vi "Metro rossa data processing.vi"() -> ()   [LabVIEW 2024]
uses:
  <vilib>/Analysis/2dsp.llb/Integral Method.ctl
  <vilib>/Analysis/8numeric.llb/1D Numeric Integration.vi
  <vilib>/Utility/file.llb/Read Delimited Spreadsheet (DBL).vi
  <vilib>/express/express analysis/Spectral/Block/exnSpectralBlock spectral measurements peak poly.vi
  <vilib>/express/express analysis/Spectral/Block/exnSpectralBlock spectral measurements peak WFM.vi
  <vilib>/express/express analysis/Spectral/Block/exnSpectralBlock spectral measurements peak DDT.vi
  <vilib>/express/express analysis/Spectral/XNode/ExpressSpectralMeasurementsBlockNode.xnode
  <vilib>/Analysis/NI_AALPro.lvlib
panel:
  out "VDV integral":dbl
  out "Angle around the choosen axis":dbl[](array[numeric])
  out "Angles":waveform(dbl)(graph)
  out "Angles in frequency domain":cluster{"f0":dbl, "df":dbl, "magnitude":dbl[]}(graph)
  out "Mean angle":dbl
  out "RMS  angle":dbl
  out "Standard Dv angle":dbl
  out "Range  angle":dbl
  in  "stop":bool
  out "Range":dbl
  out "Standard Dv":dbl
  out "RMS":dbl
  out "Mean":dbl
  out "Acceleration in frequency domain":dynamicdata(graph)
  out "Acceleration":waveform(dbl)(graph)
  out "Acceleration data extracted":dbl[](array[numeric])
  in  "choose axis":i32
  in  "Observation window length":dbl
  in  "Starting time":dbl
  out "Gyroscope":dbl[][](array[numeric])
  out "Accelerations":dbl[][](array[numeric])
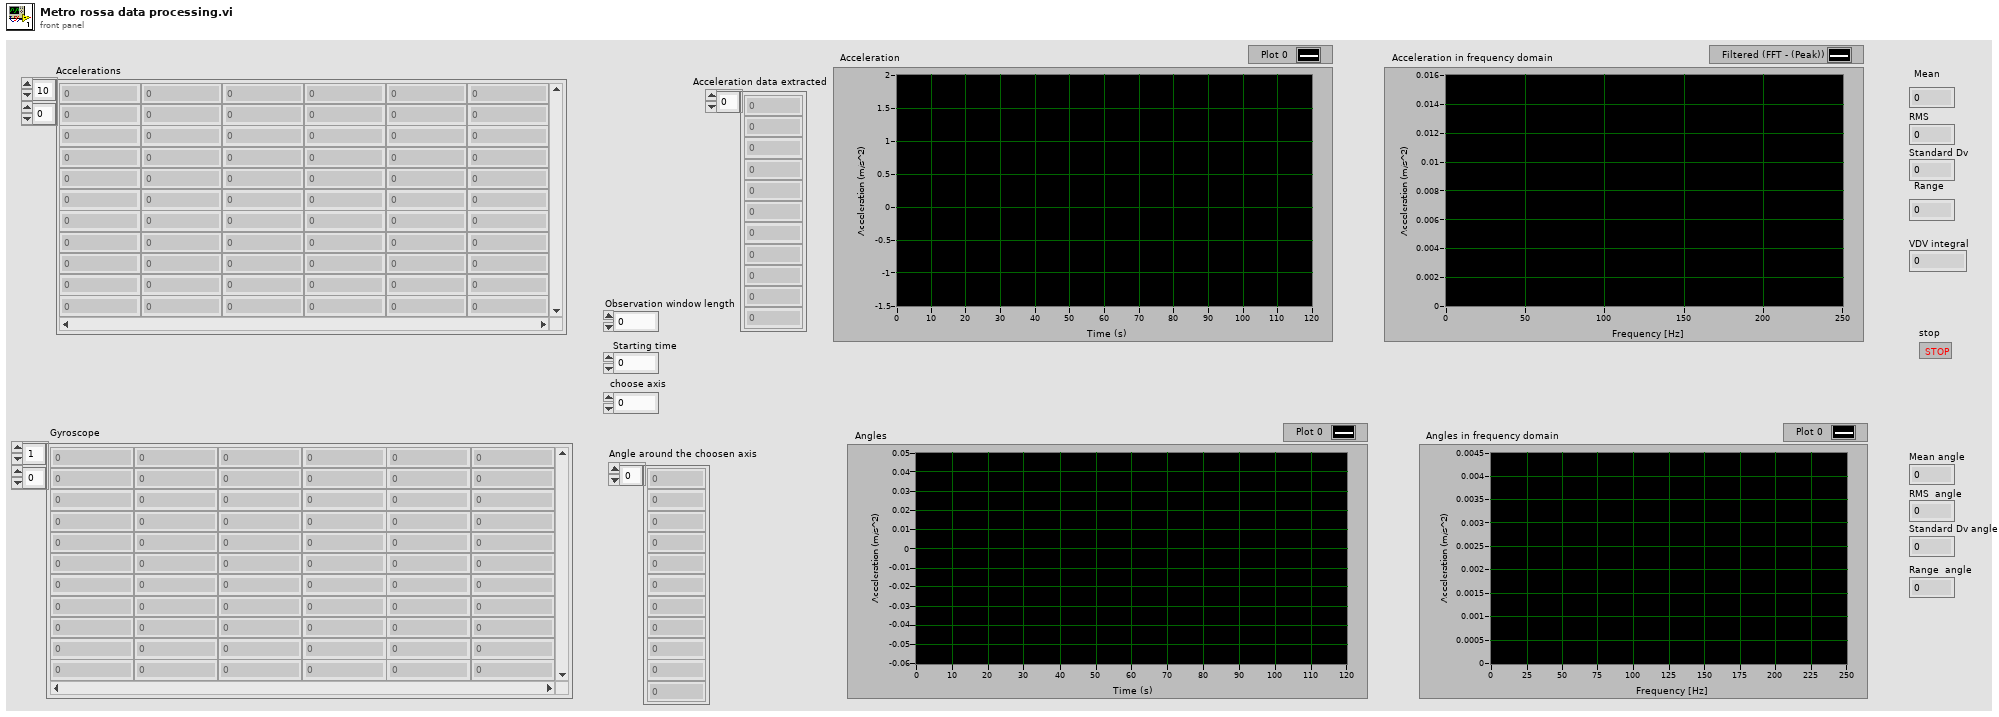
[diagram p1: front panel]
types:
  T1 = cluster{"averaging mode":u16, "weighting mode":u16, "number of averages":u32}
  T2 = cluster{"dB On (F)":bool, "unwrap phase (F)":bool, "convert to degree (F)":bool}
  T3 = typedef "NI_AALPro.lvlib/Integral Method.ctl" = i32
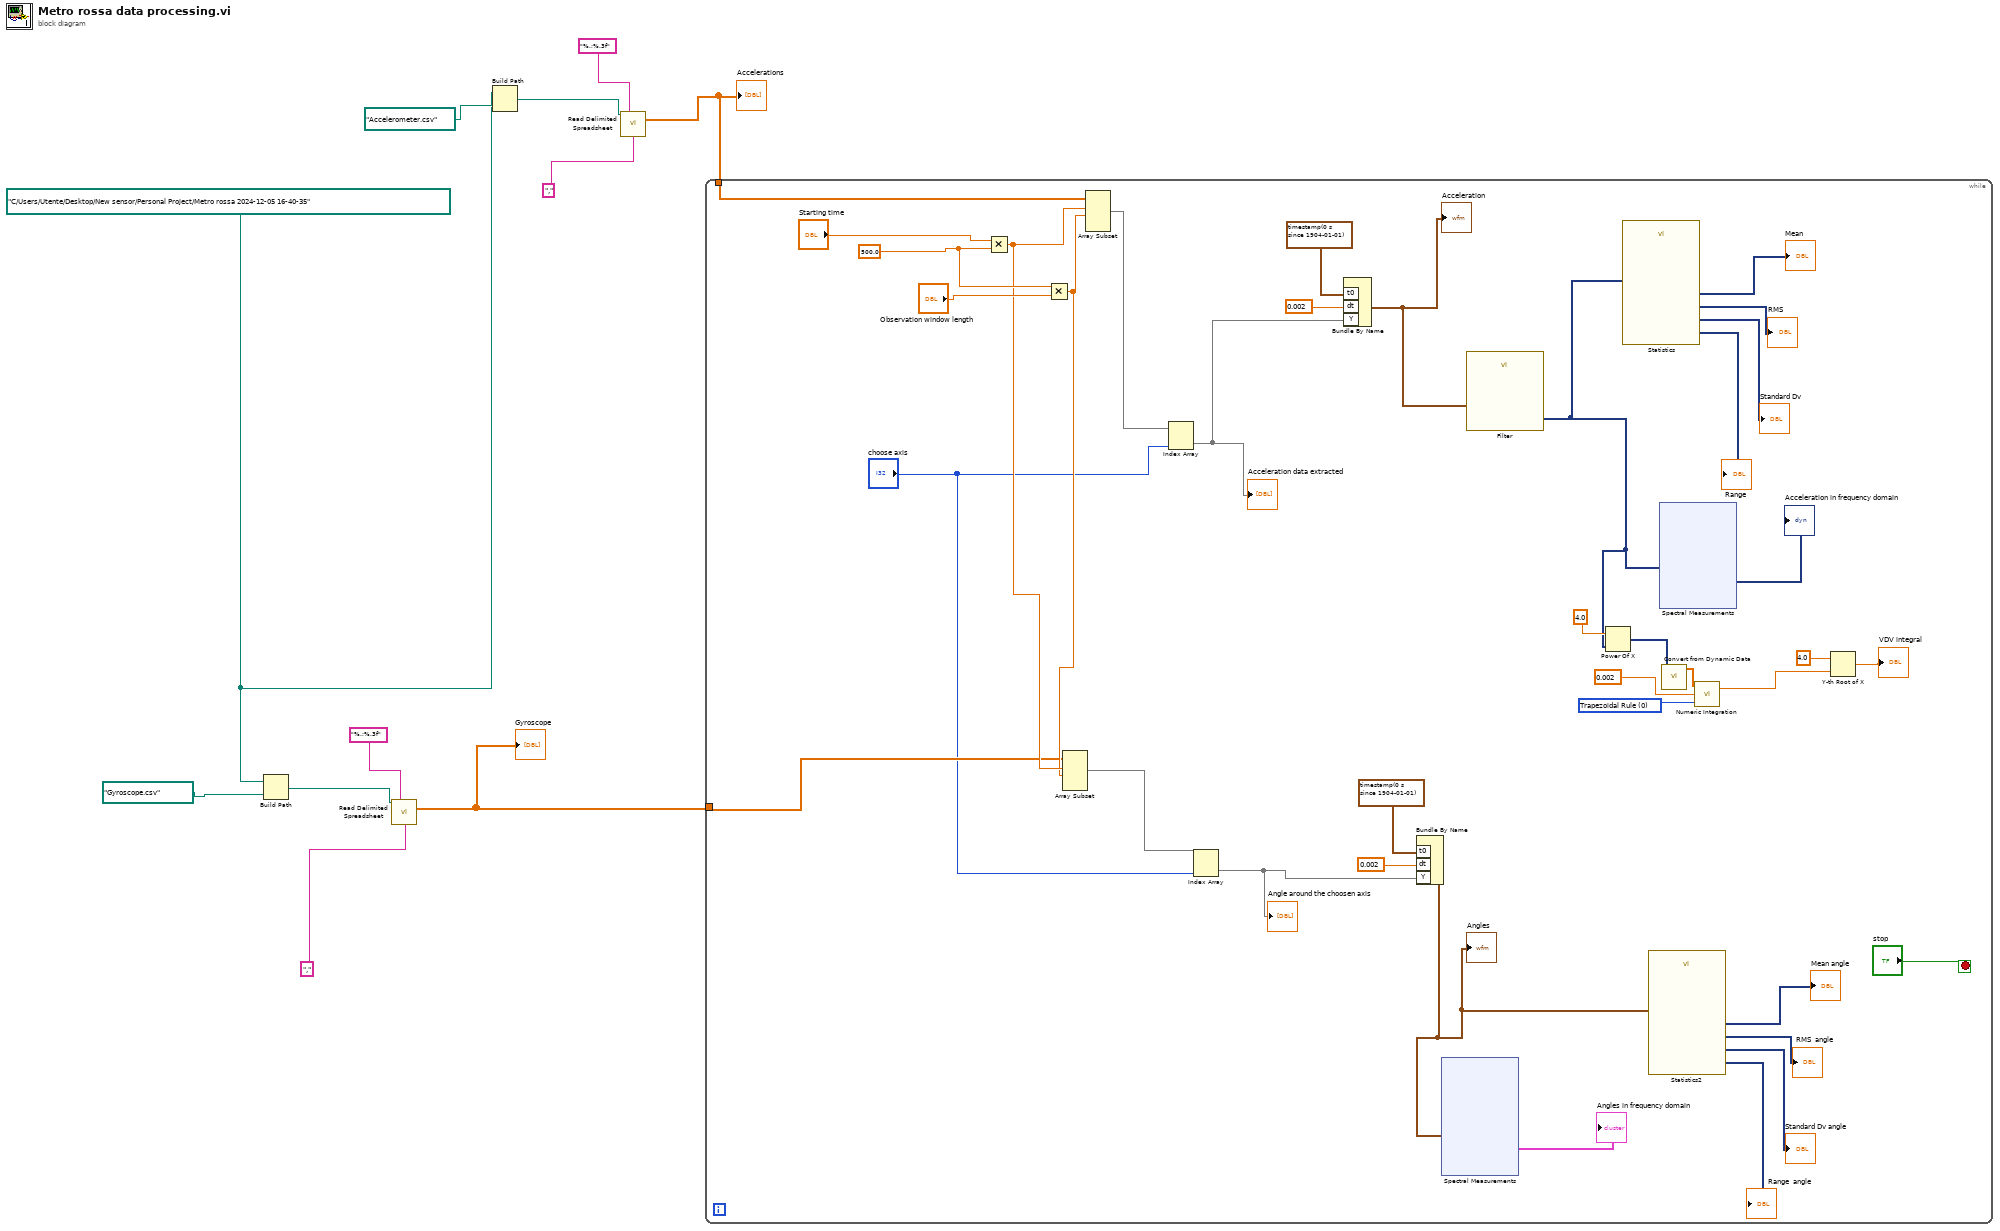
[diagram p0: block diagram]
diagram:
  w4 = path "C:/Users/Utente/Desktop/New sensor/Personal Project/Metro rossa 2024-12-05 16-40-35" ("base path")
  n1 = Build Path(base path=w4, name or relative path=path "Gyroscope.csv" ("appended path")) -> (appended path=w7:path)
  n2 = call-poly <vilib>:"Read Delimited Spreadsheet.vi"("file path (dialog if empty)"=w7, "format (%.3f)"="%.;%.3f", "delimiter (\\t)"="," ("delimiter (\\t)")) -> ("all rows"=w1:dbl[][])  [unwired: 7 in, 5 out]
  "Gyroscope" <- w1
  n3 = Build Path(base path=w4, name or relative path=path "Accelerometer.csv" ("appended path")) -> (appended path=w10:path)
  n4 = call-poly <vilib>:"Read Delimited Spreadsheet.vi"("file path (dialog if empty)"=w10, "format (%.3f)"="%.;%.3f", "delimiter (\\t)"="," ("delimiter (\\t)")) -> ("all rows"=w2:dbl[][])  [unwired: 7 in, 5 out]
  "Accelerations" <- w2
  n5 = while {
    tunnel: w2 -> [w45]
    tunnel: w1 -> [w23]
    stop <- "stop" stop-if-true
    w17 = T3 0 items=["Trapezoidal Rule", "Simpson's Rule", "Simpson's 3/8 Rule", "Bode Rule"] ("integration method")
    w48 = 500.0 ("y")
    n6 = Multiply(x="Starting time", y=w48) -> (x*y=w35:dbl)
    n7 = Multiply(x=w48, y="Observation window length") -> (x*y=w34:dbl)
    n8 = Array Subset(array=w23, index (row)=w35, length (row)=w34) -> (w26:dbl[][])  [unwired: 2 in]
    n9 = Array Subset(array=w45, index (row)=w35, length (row)=w34) -> (w46:dbl[][])  [unwired: 2 in]
    n10 = Index Array(array=w46, index (col)="choose axis") -> (element=w37:dbl[])  [unwired: 1 in]
    "Acceleration data extracted" <- w37
    n11 = Index Array(array=w26, index (col)="choose axis") -> (element=w33:dbl[])  [unwired: 1 in]
    "Angle around the choosen axis" <- w33
    n12 = Bundle By Name("t0"=timestamp(0 s since 1904-01-01), "dt"=0.002, "Y"=w37) -> (w21:waveform(dbl))  [unwired: 1 in]
    "Acceleration" <- w21
    n13 = Bundle By Name("t0"=timestamp(0 s since 1904-01-01), "dt"=0.002, "Y"=w33) -> (w32:waveform(dbl))  [unwired: 1 in]
    "Angles" <- w32
    n14 = xnode "Spectral Measurements"("Signals"=w32) -> ("FFT - (Peak)"=→"Angles in frequency domain":cluster{"f0":dbl, "df":dbl, "magnitude":dbl[]})  [unwired: 1 in, 2 out]
    n15 = call "Filter"("Signal"=w21) -> ("Filtered Signal"=w13:dynamicdata)  [unwired: 9 in, 1 out]
    n16 = Power Of X(1:w13, 2:4.0 ("y")) -> (0:w18:dynamicdata)
    n17 = call "Statistics"("Signals"=w13) -> ("Standard Dev"=→"Standard Dv":dynamicdata, "RMS"=→"RMS":dynamicdata, "Arithmetic Mean"=→"Mean":dynamicdata, "Range"=→"Range":dynamicdata)  [unwired: 22 in, 1 out]
    n18 = call "Statistics2"("Signals"=w32) -> ("Standard Dev"=→"Standard Dv angle":dynamicdata, "RMS"=→"RMS  angle":dynamicdata, "Arithmetic Mean"=→"Mean angle":dynamicdata, "Range"=→"Range  angle":dynamicdata)  [unwired: 22 in, 1 out]
    n19 = xnode "Spectral Measurements"("Signals"=w13) -> ("FFT - (Peak)"=→"Acceleration in frequency domain":dynamicdata)  [unwired: 1 in, 2 out]
    n20 = call "Convert from Dynamic Data"("Dynamic Data Type"=w18) -> ("Array"=w19:dbl[])  [unwired: 3 in]
    n21 = call-poly <vilib>:"Numeric Integration.vi"("integration method"=w17, "dt"=0.002, "Input Array"=w19) -> ("result"=w16:dbl)  [unwired: 1 out]
    n22 = Y-th Root of X(1:w16, 2:4.0 ("y")) -> (0:→"VDV integral":dbl)
  }
